vi "VI Server_Set Control Values from String Formats.vi"(6 "Options":T1, 8 "error in (no error)":errorcluster, 9 "Values":string[](array[string]), 10 "Labels":string[](array[string]), 11 "VI Server Cluster":T2={"VI Ref"=refnum, "Refs"=[], "Labels"=["Label", "Size", "Font", "Heght", "Width", "Ledding Denominator", "Ledding Nominator", "Label Number", "Microstep Resolution", "X", "Y", "Z", "Italic?", "Underlined?"]}) -> (0 "error out":errorcluster, 3 "VI Server Cluster.DUP":T2={"VI Ref"=refnum, "Refs"=[], "Labels"=["Label", "Size", "Font", "Heght", "Width", "Ledding Denominator", "Ledding Nominator", "Label Number", "Microstep Resolution", "X", "Y", "Z", "Italic?", "Underlined?"]}, 5 "FailedLabel":string)   [LabVIEW 2020, in "VI Server Toolkit LV2013.lvlib"]
doc: "<B>Set Control Values From String Formats.vi</B> and converts string values of the selected GUI objects onto original data type."
uses:
  VI Server Toolkit LV2013.lvlib
  <vilib>/userDefined/High Color/IMAQdx.ctl
  VI Server Cluster.ctl
  VI Server Libraries/VI Server Controls.llb/VI Server_GetSet Controls From String Format_Options.ctl
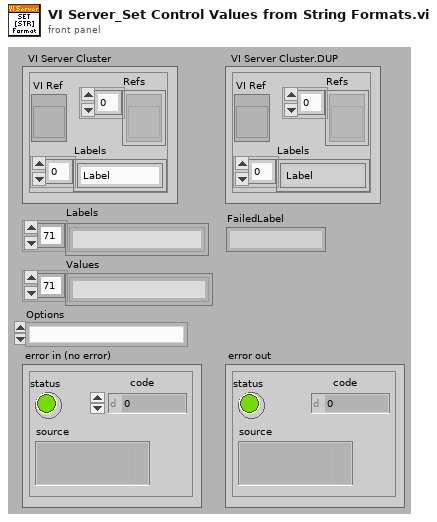
[diagram p1: front panel]
types:
  T1 = typedef "VI Server Toolkit LV2013.lvlib/VI Server_GetSet Controls From String Format_Options.ctl" = enum16{"", "If Ring Get Selection", "If Ring Set by Selection"}
  T2 = typedef "VI Server Toolkit LV2013.lvlib/VI Server Cluster.ctl" = cluster{"VI Ref":refnum<vi>, "Refs":refnum<vi>[], "Labels":string[]}
  T3 = typedef "IMAQdx.ctl" = refnum<k21>
  T4 = typedef "LVStringsAndValuesArrayTypeDef_U32.ctl" = cluster{"String":string, "Value":u32}[]
  T5 = typedef "VI Server_RefsCluster.ctl" = cluster{"Labels":string[], "Refs":refnum<vi>[], "VI Ref":refnum<vi>}
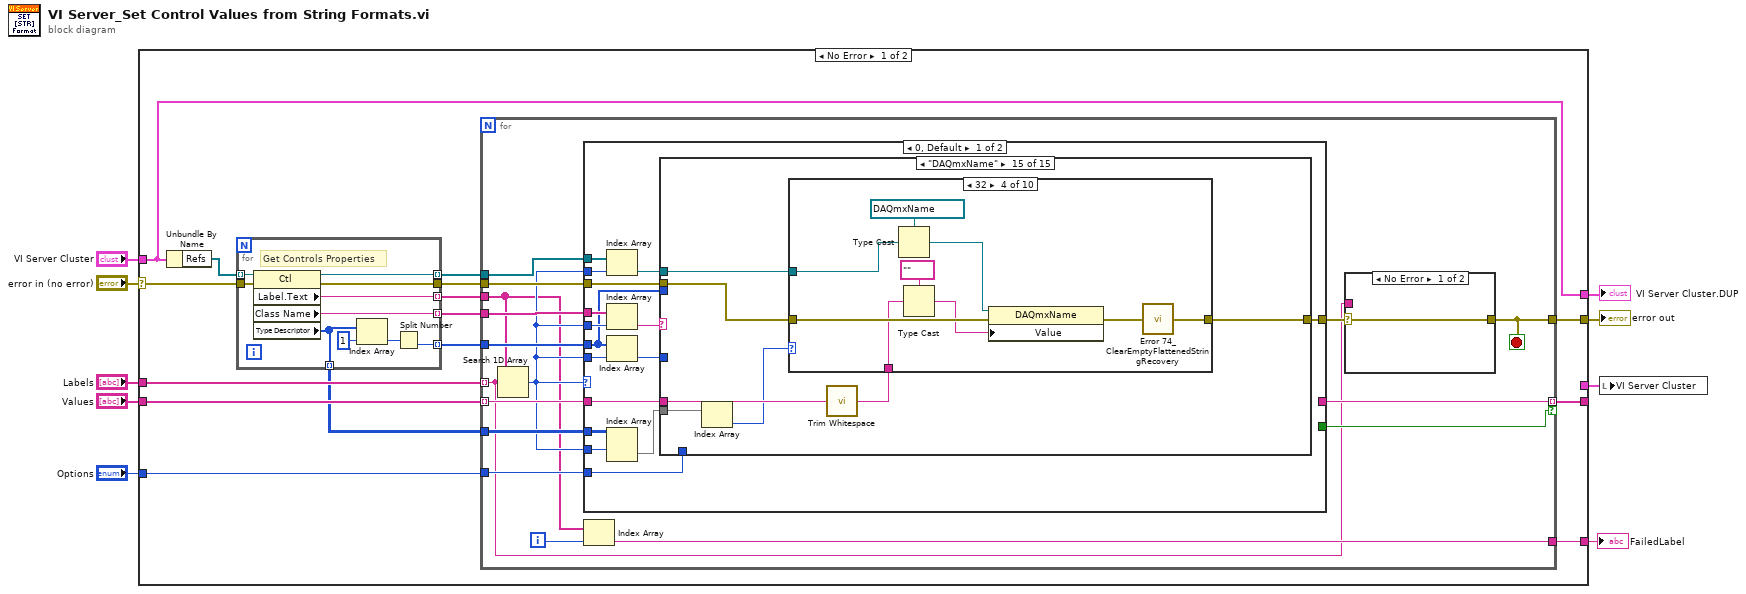
[diagram p0: block diagram]
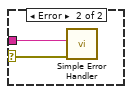
[diagram p2: hidden frame]
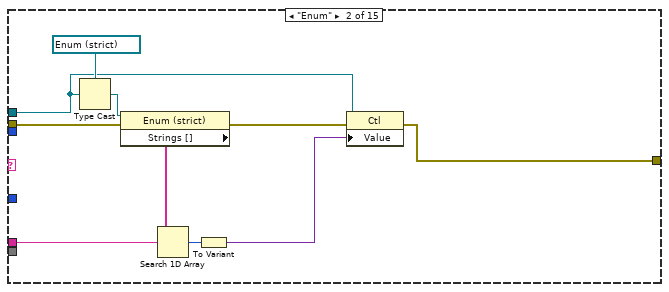
[diagram p4: hidden frame]
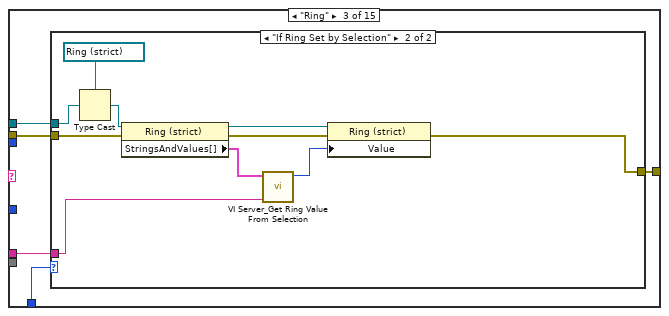
[diagram p5: hidden frame]
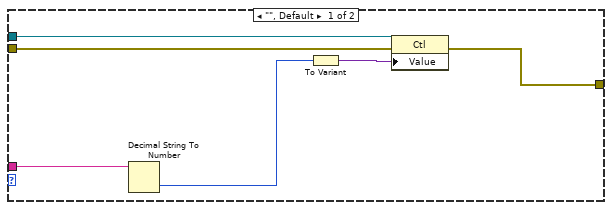
[diagram p6: hidden frame]
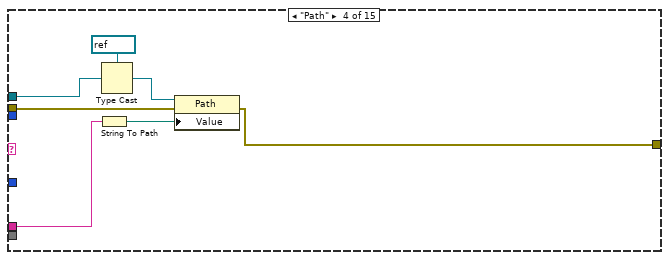
[diagram p7: hidden frame]
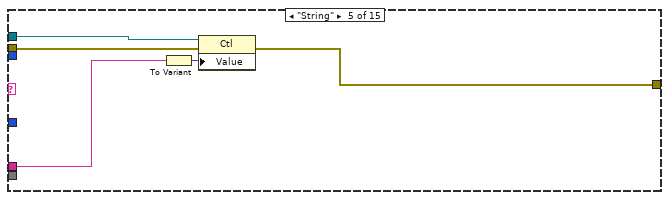
[diagram p8: hidden frame]
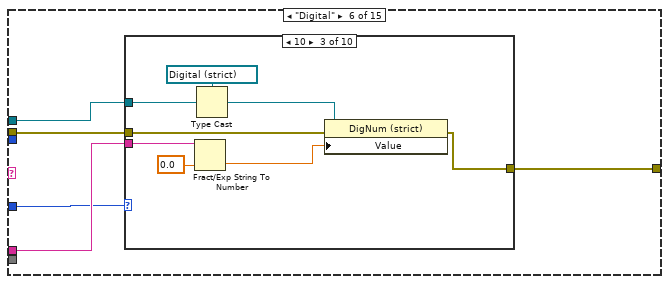
[diagram p9: hidden frame]
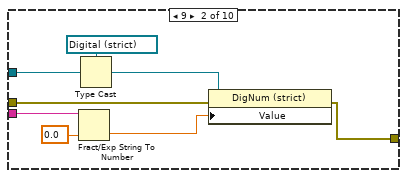
[diagram p11: hidden frame]
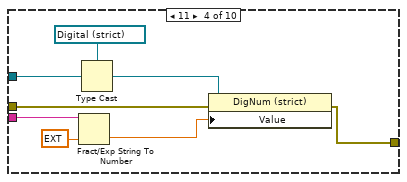
[diagram p12: hidden frame]
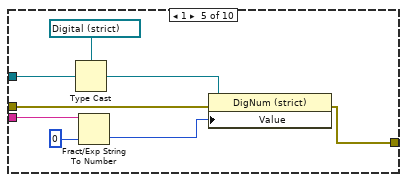
[diagram p13: hidden frame]
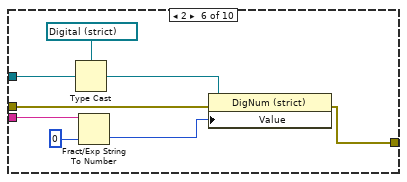
[diagram p14: hidden frame]
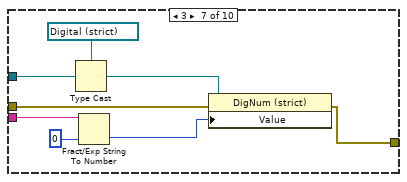
[diagram p15: hidden frame]
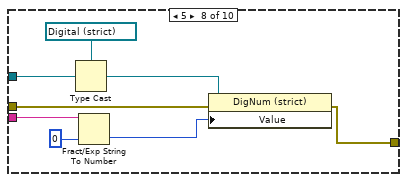
[diagram p16: hidden frame]
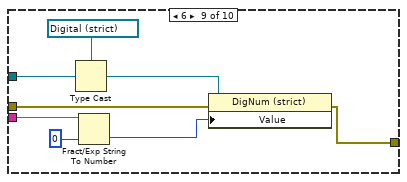
[diagram p17: hidden frame]
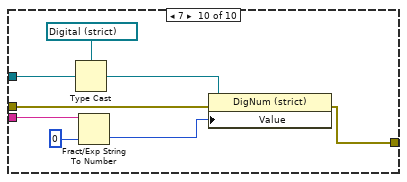
[diagram p18: hidden frame]
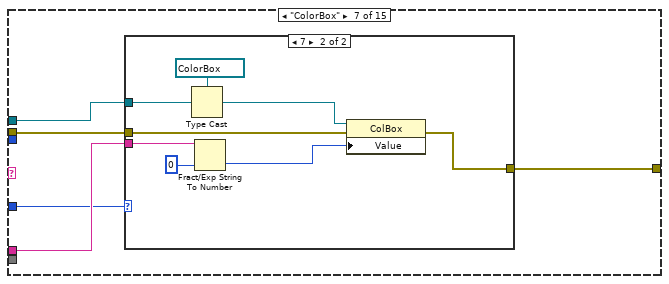
[diagram p19: hidden frame]
diagram:
  n1 = case shown="No Error" "error in (no error)" {
    selector: "error in (no error)" -> [w14 w617]
    tunnel: "Labels" -> [w19 _]
    tunnel: "Values" -> [w20 _]
    tunnel: [w13 w617] -> w7
    tunnel: [w12 _] -> w5
    tunnel: "VI Server Cluster" -> [w12 _]
    tunnel: "Options" -> [w15 _]
    tunnel: [_ w616] -> w2
    tunnel: [w11 _] -> _
    tunnel: [w10 _] -> w1
    frame No Error {
      n2 = Unbundle By Name(w12) -> ("Refs"=w18:refnum<vi>[])
      n3 = for {
        tunnel: w18 -> [w615] mode=indexing
        tunnel: w14 -> [w614]
        tunnel: [w613] -> w24 mode=indexing
        tunnel: [w612] -> w22 mode=indexing
        tunnel: [w611] -> w23 mode=indexing
        tunnel: [w610] -> w21
        tunnel: [w607] -> w17 mode=indexing
        tunnel: [w606] -> w16 mode=indexing
        # "Get Controls Properties"
        n4 = property class="Ctl"(reference=w615, error in=w614) -> (reference out=w611:refnum<vi>, error out=w610:errorcluster, "Label.Text"=w613:string, "Class Name"=w612:string, "Type Descriptor"=w606:i16[])
        n5 = Index Array(array=w606, index=1) -> (element=w608:i16)
        n6 = Split Number(x=w608) -> (lo(x)=w607:u8)  [unwired: 1 out]
      }
      n7 = for {
        tunnel: w19 -> [w25] mode=indexing
        tunnel: w24 -> [w30]
        tunnel: w23 -> [w38]
        tunnel: w22 -> [w40]
        tunnel: w20 -> [w39] mode=indexing
        tunnel: w21 -> [w37]
        tunnel: [w26] -> w13
        tunnel: w17 -> [w36]
        tunnel: w16 -> [w35]
        tunnel: w15 -> [w33]
        tunnel: [w32] -> w11 mode=indexing if=w31
        tunnel: [w28] -> w10
        i -> [w29]
        stop <- w26 stop-if-true
        n8 = Search 1D Array(1D array=w30, element=w25) -> (index of element=w34:i32)  [unwired: 1 out]
        n9 = case shown="0, Default" w34 {
          tunnel: w38 -> [w59 _]
          tunnel: w34 -> [w58 _]
          tunnel: w40 -> [w57 _]
          tunnel: w34 -> [w56 _]
          tunnel: w39 -> [w53 w604]
          tunnel: w37 -> [w52 w605]
          tunnel: [w51 w605] -> w27
          tunnel: w36 -> [w48 _]
          tunnel: w34 -> [w50 _]
          tunnel: w35 -> [w46 _]
          tunnel: w34 -> [w47 _]
          tunnel: w33 -> [w44 _]
          tunnel: [_ w604] -> w32
          tunnel: [_ TRUE] -> w31
          frame 0, Default {
            n10 = Index Array(array=w59, index=w58) -> (element=w54:refnum<vi>)
            n11 = Index Array(array=w57, index=w56) -> (element=w55:string)
            n12 = Index Array(array=w48, index=w50) -> (element=w49:u8)
            n13 = Index Array(array=w46, index (row)=w47) -> (element=w45:i16[])  [unwired: 1 in]
            n14 = case shown="\"DAQmxName\"" w55 {
              tunnel: w54 -> [_ w63 w72 w94 w103 w106 w184 w198 w288 w295 w302 w474 w496 w517 w523]
              tunnel: w53 -> [_ w68 w75 w97 w101 w105 w183 w197 w281 w293 w301 w472 w497 w518 w524]
              tunnel: w52 -> [w60 w66 w74 w95 w100 w108 w186 w200 w290 w296 w306 w476 w498 w512 w525]
              tunnel: [w60 w64 w73 w96 w99 w107 w185 w199 w289 w291 w305 w475 w495 w515 w522] -> w51
              tunnel: w49 -> [_ _ _ _ _ w104 w182 w196 _ _ _ w473 _ _ _]
              tunnel: w48 -> [_ _ _ _ _ _ _ _ _ _ _ _ _ _ _]
              tunnel: w45 -> [_ _ _ _ _ _ _ _ _ _ w304 _ _ _ w521]
              tunnel: w44 -> [_ _ w71 _ _ _ _ _ _ _ _ _ _ _ _]
              frame "", Default {
              }
              frame "Enum" {
                n15 = Type Cast(type=refnum<vi> refnum ("Enum"), x=w63) -> (*(type *) &x=w69:refnum<vi>)
                n16 = property class="Enum (strict)"(reference=w69, error in=w66) -> (error out=w65:errorcluster, "Strings []"=w67:string[])  [unwired: 1 out]
                n17 = Search 1D Array(1D array=w67, element=w68) -> (index of element=w62:i32)  [unwired: 1 out]
                n18 = To Variant(anything=w62) -> (Variant=w61:variant)
                n19 = property class="Ctl"(reference=w63, error in=w65, "Value"=w61) -> (error out=w64:errorcluster)  [unwired: 1 out]
              }
              frame "Ring" {
                n20 = case shown="\"If Ring Set by Selection\"" w71 {
                  tunnel: w75 -> [w79 w85]
                  tunnel: w74 -> [w81 w90]
                  tunnel: [w80 w88] -> w73
                  tunnel: w72 -> [w77 w87]
                  frame "", Default {
                    n21 = Decimal String To Number(string=w79) -> (number=w78:i32)  [unwired: 2 in, 1 out]
                    n22 = To Variant(anything=w78) -> (Variant=w76:variant)
                    n23 = property class="Ctl"(reference=w77, error in=w81, "Value"=w76) -> (error out=w80:errorcluster)  [unwired: 1 out]
                  }
                  frame "If Ring Set by Selection" {
                    n24 = Type Cast(type=refnum<vi> refnum ("C-867.SerialPort.Baud Rate"), x=w87) -> (*(type *) &x=w91:refnum<vi>)
                    n25 = property class="Ring (strict)"(reference=w91, error in=w90) -> (reference out=w84:refnum<vi>, error out=w89:errorcluster, "StringsAndValues[]"=w86:T4)
                    n26 = call "VI Server_Get Ring Value From Selection.vi"("Item.Selected"=w85, "StringsAndValues[]"=w86) -> ("Value"=w83:u32)  [unwired: 9 in]
                    n27 = property class="Ring (strict)"(reference=w84, error in=w89, "Value"=w83) -> (error out=w88:errorcluster)  [unwired: 1 out]
                  }
                }
              }
              frame "Path" {
                n28 = String To Path(string=w97) -> (path=w98:path)
                n29 = Type Cast(type=refnum<vi> refnum ("Path"), x=w94) -> (*(type *) &x=w93:refnum<vi>)
                n30 = property class="Path"(reference=w93, error in=w95, "Value"=w98) -> (error out=w96:errorcluster)  [unwired: 1 out]
              }
              frame "String" {
                n31 = To Variant(anything=w101) -> (Variant=w102:variant)
                n32 = property class="Ctl"(reference=w103, error in=w100, "Value"=w102) -> (error out=w99:errorcluster)  [unwired: 1 out]
              }
              frame "Digital" {
                n33 = case shown="10" w104 {
                  tunnel: w108 -> [w109 w117 w125 w133 w141 w149 w157 w165 w173 w181]
                  tunnel: [w109 w116 w124 w132 w140 w148 w156 w164 w172 w180] -> w107
                  tunnel: w106 -> [_ w115 w123 w131 w139 w147 w155 w163 w171 w179]
                  tunnel: w105 -> [_ w113 w120 w129 w137 w145 w153 w161 w169 w177]
                  frame 0, Default {
                  }
                  frame 9 {
                    n34 = Fract/Exp String To Number(string=w113, default (0 dbl)=sgl 0.0) -> (number=w112:sgl)  [unwired: 3 out]
                    n35 = Type Cast(type=refnum<vi> refnum ("SGL"), x=w115) -> (*(type *) &x=w114:refnum<vi>)
                    n36 = property class="DigNum (strict)"(reference=w114, error in=w117, "Value"=w112) -> (error out=w116:errorcluster)  [unwired: 1 out]
                  }
                  frame 10 {
                    n37 = Fract/Exp String To Number(string=w120, default (0 dbl)=0.0) -> (number=w119:dbl)  [unwired: 3 out]
                    n38 = Type Cast(type=refnum<vi> refnum ("DBL"), x=w123) -> (*(type *) &x=w121:refnum<vi>)
                    n39 = property class="DigNum (strict)"(reference=w121, error in=w125, "Value"=w119) -> (error out=w124:errorcluster)  [unwired: 1 out]
                  }
                  frame 11 {
                    n40 = Fract/Exp String To Number(string=w129, default (0 dbl)=ext 0.0) -> (number=w128:ext)  [unwired: 3 out]
                    n41 = Type Cast(type=refnum<vi> refnum ("EXT"), x=w131) -> (*(type *) &x=w130:refnum<vi>)
                    n42 = property class="DigNum (strict)"(reference=w130, error in=w133, "Value"=w128) -> (error out=w132:errorcluster)  [unwired: 1 out]
                  }
                  frame 1 {
                    n43 = Type Cast(type=refnum<vi> refnum ("I8"), x=w139) -> (*(type *) &x=w138:refnum<vi>)
                    n44 = Fract/Exp String To Number(string=w137, default (0 dbl)=i8 0) -> (number=w136:i8)  [unwired: 3 out]
                    n45 = property class="DigNum (strict)"(reference=w138, error in=w141, "Value"=w136) -> (error out=w140:errorcluster)  [unwired: 1 out]
                  }
                  frame 2 {
                    n46 = Type Cast(type=refnum<vi> refnum ("I16"), x=w147) -> (*(type *) &x=w146:refnum<vi>)
                    n47 = Fract/Exp String To Number(string=w145, default (0 dbl)=i16 0) -> (number=w144:i16)  [unwired: 3 out]
                    n48 = property class="DigNum (strict)"(reference=w146, error in=w149, "Value"=w144) -> (error out=w148:errorcluster)  [unwired: 1 out]
                  }
                  frame 3 {
                    n49 = Type Cast(type=refnum<vi> refnum ("I32"), x=w155) -> (*(type *) &x=w154:refnum<vi>)
                    n50 = Fract/Exp String To Number(string=w153, default (0 dbl)=0) -> (number=w152:i32)  [unwired: 3 out]
                    n51 = property class="DigNum (strict)"(reference=w154, error in=w157, "Value"=w152) -> (error out=w156:errorcluster)  [unwired: 1 out]
                  }
                  frame 5 {
                    n52 = Type Cast(type=refnum<vi> refnum ("U8"), x=w163) -> (*(type *) &x=w162:refnum<vi>)
                    n53 = Fract/Exp String To Number(string=w161, default (0 dbl)=u8 0) -> (number=w160:u8)  [unwired: 3 out]
                    n54 = property class="DigNum (strict)"(reference=w162, error in=w165, "Value"=w160) -> (error out=w164:errorcluster)  [unwired: 1 out]
                  }
                  frame 6 {
                    n55 = Type Cast(type=refnum<vi> refnum ("U16"), x=w171) -> (*(type *) &x=w170:refnum<vi>)
                    n56 = Fract/Exp String To Number(string=w169, default (0 dbl)=u16 0) -> (number=w168:u16)  [unwired: 3 out]
                    n57 = property class="DigNum (strict)"(reference=w170, error in=w173, "Value"=w168) -> (error out=w172:errorcluster)  [unwired: 1 out]
                  }
                  frame 7 {
                    n58 = Type Cast(type=refnum<vi> refnum ("U32"), x=w179) -> (*(type *) &x=w178:refnum<vi>)
                    n59 = Fract/Exp String To Number(string=w177, default (0 dbl)=u32 0) -> (number=w176:u32)  [unwired: 3 out]
                    n60 = property class="DigNum (strict)"(reference=w178, error in=w181, "Value"=w176) -> (error out=w180:errorcluster)  [unwired: 1 out]
                  }
                }
              }
              frame "ColorBox" {
                n61 = case shown="7" w182 {
                  tunnel: w186 -> [w187 w195]
                  tunnel: [w187 w194] -> w185
                  tunnel: w184 -> [_ w193]
                  tunnel: w183 -> [_ w191]
                  frame 0, Default {
                  }
                  frame 7 {
                    n62 = Type Cast(type=refnum<vi> refnum ("Limits.RPM.Scale.Color<=1000"), x=w193) -> (*(type *) &x=w192:refnum<vi>)
                    n63 = Fract/Exp String To Number(string=w191, default (0 dbl)=u32 0) -> (number=w190:u32)  [unwired: 3 out]
                    n64 = property class="ColBox"(reference=w192, error in=w195, "Value"=w190) -> (error out=w194:errorcluster)  [unwired: 1 out]
                  }
                }
              }
              frame "Slide" {
                n65 = case shown="7" w196 {
                  tunnel: w200 -> [w201 w209 w218 w227 w235 w243 w251 w259 w267 w275]
                  tunnel: [w201 w208 w217 w226 w234 w242 w250 w258 w266 w274] -> w199
                  tunnel: w198 -> [_ w207 w216 w225 w233 w241 w249 w257 w265 w273]
                  tunnel: w197 -> [_ w205 w213 w223 w231 w239 w247 w255 w263 w271]
                  frame 0, Default {
                  }
                  frame 9 {
                    n66 = Fract/Exp String To Number(string=w205, default (0 dbl)=sgl 0.0) -> (number=w204:sgl)  [unwired: 3 out]
                    n67 = Type Cast(type=refnum<vi> refnum ("SGL 2"), x=w207) -> (*(type *) &x=w206:refnum<vi>)
                    n68 = property class="DigNum (strict)"(reference=w206, error in=w209, "Value"=w204) -> (reference out=w210:refnum<vi>, error out=w208:errorcluster)
                    n69 = Close Reference(reference=w210) -> ()  [unwired: 1 in, 1 out]
                  }
                  frame 10 {
                    n70 = Fract/Exp String To Number(string=w213, default (0 dbl)=0.0) -> (number=w212:dbl)  [unwired: 3 out]
                    n71 = Type Cast(type=refnum<vi> refnum ("DBL 2"), x=w216) -> (*(type *) &x=w214:refnum<vi>)
                    n72 = property class="DigNum (strict)"(reference=w214, error in=w218, "Value"=w212) -> (reference out=w219:refnum<vi>, error out=w217:errorcluster)
                    n73 = Close Reference(reference=w219) -> ()  [unwired: 1 in, 1 out]
                  }
                  frame 11 {
                    n74 = Fract/Exp String To Number(string=w223, default (0 dbl)=ext 0.0) -> (number=w222:ext)  [unwired: 3 out]
                    n75 = Type Cast(type=refnum<vi> refnum ("EXT 2"), x=w225) -> (*(type *) &x=w224:refnum<vi>)
                    n76 = property class="DigNum (strict)"(reference=w224, error in=w227, "Value"=w222) -> (error out=w226:errorcluster)  [unwired: 1 out]
                  }
                  frame 1 {
                    n77 = Type Cast(type=refnum<vi> refnum ("I8 2"), x=w233) -> (*(type *) &x=w232:refnum<vi>)
                    n78 = Fract/Exp String To Number(string=w231, default (0 dbl)=i8 0) -> (number=w230:i8)  [unwired: 3 out]
                    n79 = property class="DigNum (strict)"(reference=w232, error in=w235, "Value"=w230) -> (error out=w234:errorcluster)  [unwired: 1 out]
                  }
                  frame 2 {
                    n80 = Type Cast(type=refnum<vi> refnum ("I16 2"), x=w241) -> (*(type *) &x=w240:refnum<vi>)
                    n81 = Fract/Exp String To Number(string=w239, default (0 dbl)=i16 0) -> (number=w238:i16)  [unwired: 3 out]
                    n82 = property class="DigNum (strict)"(reference=w240, error in=w243, "Value"=w238) -> (error out=w242:errorcluster)  [unwired: 1 out]
                  }
                  frame 3 {
                    n83 = Type Cast(type=refnum<vi> refnum ("I32 2"), x=w249) -> (*(type *) &x=w248:refnum<vi>)
                    n84 = Fract/Exp String To Number(string=w247, default (0 dbl)=0) -> (number=w246:i32)  [unwired: 3 out]
                    n85 = property class="DigNum (strict)"(reference=w248, error in=w251, "Value"=w246) -> (error out=w250:errorcluster)  [unwired: 1 out]
                  }
                  frame 5 {
                    n86 = Type Cast(type=refnum<vi> refnum ("U8 2"), x=w257) -> (*(type *) &x=w256:refnum<vi>)
                    n87 = Fract/Exp String To Number(string=w255, default (0 dbl)=u8 0) -> (number=w254:u8)  [unwired: 3 out]
                    n88 = property class="DigNum (strict)"(reference=w256, error in=w259, "Value"=w254) -> (error out=w258:errorcluster)  [unwired: 1 out]
                  }
                  frame 6 {
                    n89 = Type Cast(type=refnum<vi> refnum ("U16 2"), x=w265) -> (*(type *) &x=w264:refnum<vi>)
                    n90 = Fract/Exp String To Number(string=w263, default (0 dbl)=u16 0) -> (number=w262:u16)  [unwired: 3 out]
                    n91 = property class="DigNum (strict)"(reference=w264, error in=w267, "Value"=w262) -> (error out=w266:errorcluster)  [unwired: 1 out]
                  }
                  frame 7 {
                    n92 = Type Cast(type=refnum<vi> refnum ("U32 2"), x=w273) -> (*(type *) &x=w272:refnum<vi>)
                    n93 = Fract/Exp String To Number(string=w271, default (0 dbl)=u32 0) -> (number=w270:u32)  [unwired: 3 out]
                    n94 = property class="DigNum (strict)"(reference=w272, error in=w275, "Value"=w270) -> (error out=w274:errorcluster)  [unwired: 1 out]
                  }
                }
              }
              frame "Boolean" {
                n95 = Type Cast(type=refnum<vi> refnum ("Boolean"), x=w288) -> (*(type *) &x=w286:refnum<vi>)
                n96 = Equal?(x=w281, y="TRUE" ("x")) -> (x = y?=w284:bool)
                n97 = Equal?(x=w281, y="ON" ("x")) -> (x = y?=w280:bool)
                n98 = Equal?(x=w281, y="1" ("x")) -> (x = y?=w279:bool)
                n99 = Compound Arithmetic op=OR(w284, w280, w279) -> (w278:bool)
                n100 = Type Cast(type=FALSE ("Value"), x=w278) -> (*(type *) &x=w276:bool)
                n101 = property class="Bool (strict)"(reference=w286, error in=w290, "Value"=w276) -> (error out=w289:errorcluster)  [unwired: 1 out]
              }
              frame "Table" {
                n102 = Type Cast(type=refnum<vi> refnum ("Image Statistics Table"), x=w295) -> (*(type *) &x=w298:refnum<vi>)
                n103 = Spreadsheet String To Array(delimiter (Tab)=",", format string="%s", spreadsheet string=w293, array type (2D Dbl)=string[][] []) -> (array=w292:string[][])
                n104 = property class="Tbl (strict)"(reference=w298, error in=w296, "Value"=w292) -> (error out=w291:errorcluster)  [unwired: 1 out]
              }
              frame "Array" {
                n105 = Index Array(array=w304, index=2) -> (element=w303:i16)
                n106 = case shown="1" w303 {
                  tunnel: w304 -> [_ w314 w356]
                  tunnel: w306 -> [w308 w313 w355]
                  tunnel: [w308 w311 w354] -> w305
                  tunnel: w302 -> [_ w310 w353]
                  tunnel: w301 -> [_ w309 w352]
                  frame 0, Default {
                  }
                  frame 1 {
                    # "1D Array\ndata Type"
                    n107 = Index Array(array=w314, index=6) -> (element=w312:i16)
                    n108 = case shown="4032" w312 {
                      tunnel: w310 -> [_ w326 w336 w347]
                      tunnel: [w316 w324 w334 w345] -> w311
                      tunnel: w313 -> [w316 w323 w333 w344]
                      tunnel: w309 -> [_ w319 w329 w342]
                      frame 0, Default {
                      }
                      frame 16394 {
                        n109 = Spreadsheet String To Array(delimiter (Tab)=",", format string="%0.6f", spreadsheet string=w319, array type (2D Dbl)=dbl[] []) -> (array=w317:dbl[])
                        n110 = Type Cast(type=refnum<vi> refnum ("Array"), x=w326) -> (*(type *) &x=w325:refnum<vi>)
                        n111 = property class="Arr (strict)"(reference=w325, error in=w323, "Value"=w317) -> (error out=w324:errorcluster)  [unwired: 1 out]
                      }
                      frame 16432 {
                        n112 = Spreadsheet String To Array(delimiter (Tab)=",", format string="%s", spreadsheet string=w329, array type (2D Dbl)=string[] []) -> (array=w327:string[])
                        n113 = Type Cast(type=refnum<vi> refnum ("1D String"), x=w336) -> (*(type *) &x=w335:refnum<vi>)
                        n114 = property class="Arr (strict)"(reference=w335, error in=w333, "Value"=w327) -> (error out=w334:errorcluster)  [unwired: 1 out]
                      }
                      frame 16434 {
                        n115 = Spreadsheet String To Array(delimiter (Tab)=",", format string="%s", spreadsheet string=w342, array type (2D Dbl)=string[] []) -> (array=w338:string[])
                        n116 = for {
                          tunnel: w338 -> [w349] mode=indexing
                          tunnel: [w348] -> w337 mode=indexing
                          n117 = String To Path(string=w349) -> (path=w348:path)
                        }
                        n118 = Type Cast(type=refnum<vi> refnum ("Array"), x=w347) -> (*(type *) &x=w346:refnum<vi>)
                        n119 = property class="Arr (strict)"(reference=w346, error in=w344, "Value"=w337) -> (error out=w345:errorcluster)  [unwired: 1 out]
                      }
                    }
                  }
                  frame 2 {
                    n120 = Index Array(array=w356, index=8) -> (element=w351:i16)
                    n121 = Split Number(x=w351) -> (lo(x)=w350:u8)  [unwired: 1 out]
                    n122 = case shown="32" w350 {
                      tunnel: w353 -> [_ w368 w378 w388 w398 w408 w418 w428 w438 w448 w458 w469]
                      tunnel: [w358 w366 w376 w386 w396 w406 w416 w426 w436 w446 w456 w467] -> w354
                      tunnel: w355 -> [w358 w365 w375 w385 w395 w405 w415 w425 w435 w445 w455 w466]
                      tunnel: w352 -> [_ w362 w372 w382 w392 w402 w412 w422 w432 w442 w452 w465]
                      frame 0, Default {
                      }
                      frame 1 {
                        n123 = Spreadsheet String To Array(delimiter (Tab)=",", format string="%d", spreadsheet string=w362, array type (2D Dbl)=i8[][] []) -> (array=w360:i8[][])
                        n124 = Type Cast(type=refnum<vi> refnum ("Array"), x=w368) -> (*(type *) &x=w367:refnum<vi>)
                        n125 = property class="Arr (strict)"(reference=w367, error in=w365, "Value"=w360) -> (error out=w366:errorcluster)  [unwired: 1 out]
                      }
                      frame 2 {
                        n126 = Spreadsheet String To Array(delimiter (Tab)=",", format string="%d", spreadsheet string=w372, array type (2D Dbl)=i16[][] []) -> (array=w370:i16[][])
                        n127 = Type Cast(type=refnum<vi> refnum ("Array"), x=w378) -> (*(type *) &x=w377:refnum<vi>)
                        n128 = property class="Arr (strict)"(reference=w377, error in=w375, "Value"=w370) -> (error out=w376:errorcluster)  [unwired: 1 out]
                      }
                      frame 3 {
                        n129 = Spreadsheet String To Array(delimiter (Tab)=",", format string="%d", spreadsheet string=w382, array type (2D Dbl)=i32[][] []) -> (array=w380:i32[][])
                        n130 = Type Cast(type=refnum<vi> refnum ("Array"), x=w388) -> (*(type *) &x=w387:refnum<vi>)
                        n131 = property class="Arr (strict)"(reference=w387, error in=w385, "Value"=w380) -> (error out=w386:errorcluster)  [unwired: 1 out]
                      }
                      frame 5 {
                        n132 = Spreadsheet String To Array(delimiter (Tab)=",", format string="%d", spreadsheet string=w392, array type (2D Dbl)=u8[][] []) -> (array=w390:u8[][])
                        n133 = Type Cast(type=refnum<vi> refnum ("Array"), x=w398) -> (*(type *) &x=w397:refnum<vi>)
                        n134 = property class="Arr (strict)"(reference=w397, error in=w395, "Value"=w390) -> (error out=w396:errorcluster)  [unwired: 1 out]
                      }
                      frame 6 {
                        n135 = Spreadsheet String To Array(delimiter (Tab)=",", format string="%d", spreadsheet string=w402, array type (2D Dbl)=u16[][] []) -> (array=w400:u16[][])
                        n136 = Type Cast(type=refnum<vi> refnum ("Array"), x=w408) -> (*(type *) &x=w407:refnum<vi>)
                        n137 = property class="Arr (strict)"(reference=w407, error in=w405, "Value"=w400) -> (error out=w406:errorcluster)  [unwired: 1 out]
                      }
                      frame 7 {
                        n138 = Spreadsheet String To Array(delimiter (Tab)=",", format string="%d", spreadsheet string=w412, array type (2D Dbl)=u32[][] []) -> (array=w410:u32[][])
                        n139 = Type Cast(type=refnum<vi> refnum ("Array"), x=w418) -> (*(type *) &x=w417:refnum<vi>)
                        n140 = property class="Arr (strict)"(reference=w417, error in=w415, "Value"=w410) -> (error out=w416:errorcluster)  [unwired: 1 out]
                      }
                      frame 9 {
                        n141 = Spreadsheet String To Array(delimiter (Tab)=",", format string="%f", spreadsheet string=w422, array type (2D Dbl)=sgl[][] []) -> (array=w420:sgl[][])
                        n142 = Type Cast(type=refnum<vi> refnum ("Array"), x=w428) -> (*(type *) &x=w427:refnum<vi>)
                        n143 = property class="Arr (strict)"(reference=w427, error in=w425, "Value"=w420) -> (error out=w426:errorcluster)  [unwired: 1 out]
                      }
                      frame 10 {
                        n144 = Spreadsheet String To Array(delimiter (Tab)=",", format string="%f", spreadsheet string=w432, array type (2D Dbl)=dbl[][] []) -> (array=w430:dbl[][])
                        n145 = Type Cast(type=refnum<vi> refnum ("Array"), x=w438) -> (*(type *) &x=w437:refnum<vi>)
                        n146 = property class="Arr (strict)"(reference=w437, error in=w435, "Value"=w430) -> (error out=w436:errorcluster)  [unwired: 1 out]
                      }
                      frame 11 {
                        n147 = Spreadsheet String To Array(delimiter (Tab)=",", format string="%f", spreadsheet string=w442, array type (2D Dbl)=ext[][] []) -> (array=w440:ext[][])
                        n148 = Type Cast(type=refnum<vi> refnum ("Array"), x=w448) -> (*(type *) &x=w447:refnum<vi>)
                        n149 = property class="Arr (strict)"(reference=w447, error in=w445, "Value"=w440) -> (error out=w446:errorcluster)  [unwired: 1 out]
                      }
                      frame 48 {
                        n150 = Spreadsheet String To Array(delimiter (Tab)=",", format string="%s", spreadsheet string=w452, array type (2D Dbl)=string[][] []) -> (array=w450:string[][])
                        n151 = Type Cast(type=refnum<vi> refnum ("Array"), x=w458) -> (*(type *) &x=w457:refnum<vi>)
                        n152 = property class="Arr (strict)"(reference=w457, error in=w455, "Value"=w450) -> (error out=w456:errorcluster)  [unwired: 1 out]
                      }
                      frame 50 {
                        n153 = Spreadsheet String To Array(delimiter (Tab)=",", format string="%s", spreadsheet string=w465, array type (2D Dbl)=string[][] []) -> (array=w461:string[][])
                        n154 = for {
                          tunnel: w461 -> [w471] mode=indexing
                          tunnel: [w470] -> w460 mode=indexing
                          n155 = String To Path(string=w471) -> (path=w470:path[])
                        }
                        n156 = Type Cast(type=refnum<vi> refnum ("Array"), x=w469) -> (*(type *) &x=w468:refnum<vi>)
                        n157 = property class="Arr (strict)"(reference=w468, error in=w466, "Value"=w460) -> (error out=w467:errorcluster)  [unwired: 1 out]
                      }
                    }
                  }
                }
              }
              frame "MulticolumnListbox" {
                n158 = case shown="3" w473 {
                  tunnel: w476 -> [w477 w482 w493]
                  tunnel: [w477 w481 w492] -> w475
                  tunnel: w474 -> [_ w484 w494]
                  tunnel: w472 -> [_ w479 w489]
                  frame 0, Default {
                  }
                  frame 3 {
                    n159 = Decimal String To Number(string=w479) -> (number=w478:i32)  [unwired: 2 in, 1 out]
                    n160 = Type Cast(type=refnum<vi> refnum ("Controls Description"), x=w484) -> (*(type *) &x=w480:refnum<vi>)
                    n161 = property class="MCListbox (strict)"(reference=w480, error in=w482, "Value"=w478) -> (error out=w481:errorcluster)  [unwired: 1 out]
                  }
                  frame 64 {
                    n162 = Spreadsheet String To Array(delimiter (Tab)=",", format string="%s", spreadsheet string=w489, array type (2D Dbl)=i32[] [] ("Value")) -> (array=w485:i32[])
                    n163 = Type Cast(type=refnum<vi> refnum ("Controls Description"), x=w494) -> (*(type *) &x=w491:refnum<vi>)
                    n164 = property class="MCListbox (strict)"(reference=w491, error in=w493, "Value"=w485) -> (error out=w492:errorcluster)  [unwired: 1 out]
                  }
                }
              }
              frame "GenClassTagRef" {
                n165 = disable-structure shown="Disabled" {
                  disable-tunnel: w498 -> [w508 w509]
                  disable-tunnel: w497 -> [w507 _]
                  disable-tunnel: w496 -> [w505 _]
                  disable-tunnel: [w500 w509] -> w495
                  frame Disabled {
                    n166 = Type Cast(type=refnum<vi> refnum ("Camera.Left"), x=w505) -> (*(type *) &x=w502:refnum<vi>)
                    n167 = Unflatten From String(type=T3 refnum ("Camera.Left"), binary string=w507, error in (no error)=w508) -> (value=w501:T3, error out=w503:errorcluster)  [unwired: 2 in, 1 out]
                    n168 = property class="IMAQdx (strict)"(reference=w502, error in=w503, "Value"=w501) -> (error out=w499:errorcluster)  [unwired: 1 out]
                    n169 = call <vilib>:"Simple Error Handler.vi"("error in (no error)"=w499) -> ()  [unwired: 4 in, 5 out]
                    n170 = call "Error 74_ClearEmptyFlattenedStringRecovery.vi"("error in"=w499) -> ("error out"=w500:errorcluster)  [unwired: 3 in, 1 out]
                  }
                  frame Enabled {
                  }
                }
              }
              frame "VISAResourceName" {
                n171 = call <vilib>:"Trim Whitespace.vi"("string"=w518) -> ("trimmed string"=w511:string)  [unwired: 1 in]
                n172 = Type Cast(type=refnum<vi> refnum ("VISA resource name"), x=w517) -> (*(type *) &x=w516:refnum<vi>)
                n173 = Type Cast(type=refnum<visa-resource-name> refnum ("GPS.VISA.ResourceName"), x=w511) -> (*(type *) &x=w510:refnum<visa-resource-name>)
                n174 = property class="VISAName"(reference=w516, error in=w512, "Value"=w510) -> (error out=w515:errorcluster)  [unwired: 1 out]
              }
              frame "DAQmxName" {
                n175 = Index Array(array=w521) -> (element=w520:i16)  [unwired: 1 in]
                n176 = call <vilib>:"Trim Whitespace.vi"("string"=w524) -> ("trimmed string"=w519:string)  [unwired: 1 in]
                n177 = case shown="32" w520 {
                  tunnel: w525 -> [w526 w530 w539 w548 w557 w563 w575 w582 w587 w597]
                  tunnel: w519 -> [_ w528 w538 w546 w555 w565 w574 w581 w590 w599]
                  tunnel: w523 -> [_ w535 w544 w553 w562 w570 w578 w586 w594 w602]
                  tunnel: [w526 w531 w540 w550 w559 w569 w577 w585 w592 w601] -> w522
                  frame 0, Default {
                  }
                  frame 26, 38 {
                    n178 = Type Cast(type=refnum<vi> refnum ("CamTriggerGenerator.Counter"), x=w535) -> (*(type *) &x=w534:refnum<vi>)
                    n179 = Type Cast(type=tag "" ("CamTriggerGenerator.Counter"), x=w528) -> (*(type *) &x=w527:tag)
                    n180 = property class="DAQmxName"(reference=w534, error in=w530, "Value"=w527) -> (error out=w532:errorcluster)  [unwired: 1 out]
                    n181 = call "Error 74_ClearEmptyFlattenedStringRecovery.vi"("error in"=w532) -> ("error out"=w531:errorcluster)  [unwired: 3 in, 1 out]
                  }
                  frame 30 {
                    n182 = Type Cast(type=refnum<vi> refnum ("CamTriggerGenerator.Counter"), x=w544) -> (*(type *) &x=w543:refnum<vi>)
                    n183 = Type Cast(type=tag "Dev2/port1/line3" ("DAQ.GPM.DigitalLine"), x=w538) -> (*(type *) &x=w537:tag)
                    n184 = property class="DAQmxName"(reference=w543, error in=w539, "Value"=w537) -> (error out=w541:errorcluster)  [unwired: 1 out]
                    n185 = call "Error 74_ClearEmptyFlattenedStringRecovery.vi"("error in"=w541) -> ("error out"=w540:errorcluster)  [unwired: 3 in, 1 out]
                  }
                  frame 32 {
                    n186 = Type Cast(type=refnum<vi> refnum ("DAQmx.Digital Output"), x=w553) -> (*(type *) &x=w552:refnum<vi>)
                    n187 = Type Cast(type=tag "" ("DAQmx.Digital Output"), x=w546) -> (*(type *) &x=w547:tag)
                    n188 = property class="DAQmxName"(reference=w552, error in=w548, "Value"=w547) -> (error out=w551:errorcluster)  [unwired: 1 out]
                    n189 = call "Error 74_ClearEmptyFlattenedStringRecovery.vi"("error in"=w551) -> ("error out"=w550:errorcluster)  [unwired: 3 in, 1 out]
                  }
                  frame 34 {
                    n190 = Type Cast(type=refnum<vi> refnum ("DAQmx.Digital Output"), x=w562) -> (*(type *) &x=w561:refnum<vi>)
                    n191 = Type Cast(type=tag "Dev2/ai1" ("DAQ.EngineTilt.Channel"), x=w555) -> (*(type *) &x=w556:tag)
                    n192 = property class="DAQmxName"(reference=w561, error in=w557, "Value"=w556) -> (error out=w560:errorcluster)  [unwired: 1 out]
                    n193 = call "Error 74_ClearEmptyFlattenedStringRecovery.vi"("error in"=w560) -> ("error out"=w559:errorcluster)  [unwired: 3 in, 1 out]
                  }
                  frame 40 {
                    n194 = Type Cast(type=refnum<vi> refnum ("IlluminationControl.DigitalLines"), x=w570) -> (*(type *) &x=w568:refnum<vi>)
                    n195 = Type Cast(type=tag "Dev1/ctr0" ("Engine.FuelPump.DAQmx.Counter"), x=w565) -> (*(type *) &x=w564:tag)
                    n196 = property class="DAQmxName"(reference=w568, error in=w563, "Value"=w564) -> (error out=w569:errorcluster)  [unwired: 1 out]
                  }
                  frame 42, 48 {
                    n197 = Type Cast(type=refnum<vi> refnum ("Engine.FuelPump.PauseTrigger.DO"), x=w578) -> (*(type *) &x=w576:refnum<vi>)
                    n198 = Type Cast(type=tag "Dev1/port0/line7" ("Engine.FuelPump.PauseTrigger.DO"), x=w574) -> (*(type *) &x=w572:tag)
                    n199 = property class="DAQmxName"(reference=w576, error in=w575, "Value"=w572) -> (error out=w577:errorcluster)  [unwired: 1 out]
                  }
                  frame 44 {
                    n200 = Type Cast(type=refnum<vi> refnum ("IlluminationControl.DigitalLines"), x=w586) -> (*(type *) &x=w584:refnum<vi>)
                    n201 = Type Cast(type=tag "Dev2/port0/line0:1" ("IlluminationControl.DigitalLines"), x=w581) -> (*(type *) &x=w580:tag)
                    n202 = property class="DAQmxName"(reference=w584, error in=w582, "Value"=w580) -> (error out=w585:errorcluster)  [unwired: 1 out]
                  }
                  frame 46 {
                    n203 = Type Cast(type=refnum<vi> refnum ("Engine.FuelPump.PauseTriggerSource"), x=w594) -> (*(type *) &x=w593:refnum<vi>)
                    n204 = Type Cast(type=tag "Output Terminal" ("CamTriggerGenerator.OutputTerminal"), x=w590) -> (*(type *) &x=w588:tag)
                    n205 = property class="DAQmxName"(reference=w593, error in=w587, "Value"=w588) -> (error out=w592:errorcluster)  [unwired: 1 out]
                  }
                  frame 50 {
                    n206 = Type Cast(type=refnum<vi> refnum ("DAQmx.RPM.FrequencyMonitor.DigitalLine"), x=w602) -> (*(type *) &x=w600:refnum<vi>)
                    n207 = Type Cast(type=tag "" ("DAQmx.RPM.FrequencyMonitor.DigitalLine"), x=w599) -> (*(type *) &x=w598:tag)
                    n208 = property class="DAQmxName"(reference=w600, error in=w597, "Value"=w598) -> (error out=w601:errorcluster)  [unwired: 1 out]
                  }
                }
              }
            }
          }
          frame -1 {
          }
        }
        n209 = Index Array(array=w30, index=w29) -> (element=w28:string)
        n210 = case shown="No Error" w27 {
          selector: w27 -> [w41 w43]
          tunnel: [w41 _] -> w26
          tunnel: w25 -> [_ w42]
          frame No Error {
          }
          frame Error {
            n211 = call <vilib>:"Simple Error Handler.vi"("error source (\" \")"=w42, "error in (no error)"=w43) -> ()  [unwired: 3 in, 5 out]
          }
        }
      }
    }
    frame Error {
      n212 = call "VI Server_Empty VI Server Cluster.vi"() -> ("VI Server Cluster"=w616:T5)  [unwired: 7 in]
    }
  }
  "error out" <- w7
  "VI Server Cluster.DUP" <- w5
  "FailedLabel" <- w1
  n213 = local write "VI Server Cluster"(w2) -> ()
